vi "Goal_get.vi"(8 "error in (no error)":errorcluster) -> (0 "error out":errorcluster, 2 "Goal":cluster{"X":dbl, "Y":dbl})   [LabVIEW 2009, in "NetworkVarTarget.lvlib"]
uses:
  NetworkVarTarget.lvlib
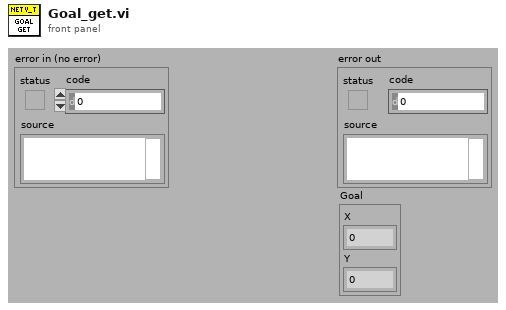
[diagram p1: front panel]
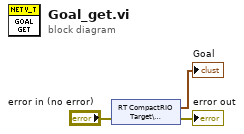
[diagram p0: block diagram]
diagram:
  n1 = shared-variable "RT CompactRIO Target\\NetworkVar.lvlib\\Goal"(error in="error in (no error)") -> (→"Goal":cluster{"X":dbl, "Y":dbl}, error out=→"error out":errorcluster)
